vi "Path2PathSup.vi"(8 "Jump Speed":dbl, 9 "Mark Speed":dbl, 10 "Power":dbl, 11 "Combined":T2) -> (3 "PathSupreme":T3)   [LabVIEW 2014]
uses:
  TypeDefs/PathSupreme.ctl
  PBFAM/Controller/MachineController/Converters/ScanSub/VelocityProfile.ctl
  PBFAM/Controller/MachineController/Converters/ScanSub/PathCut.ctl
  PBFAM/Controller/MachineController/Converters/ScanSub/Segment.ctl
  TypeDefs/Point2DwSlope.ctl
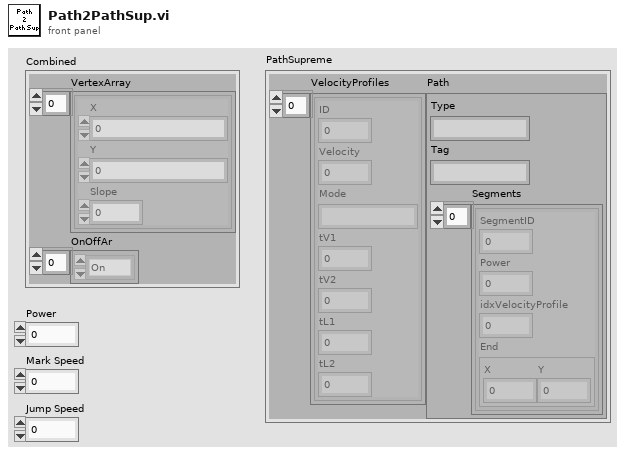
[diagram p1: front panel]
types:
  T1 = typedef "Point2DwSlope.ctl" = cluster{"X":sgl, "Y":sgl, "Slope":dbl}
  T2 = cluster{"VertexArray":T1[], "OnOffAr":enum16{"On", "Off"}[]}
  T3 = typedef "PathSupreme.ctl" = cluster{"VelocityProfiles":T4[], "Path":T5}
  T4 = typedef "VelocityProfile.ctl" = cluster{"ID":u32, "Velocity":dbl, "Mode":string, "tV1":u32, "tV2":u32, "tL1":u32, "tL2":u32}
  T5 = typedef "PathCut.ctl" = cluster{"Type":string, "Tag":string, "Segments":T6[]}
  T6 = typedef "Segment.ctl" = cluster{"SegmentID":u16, "Power":sgl, "idxVelocityProfile":u16, "End":cluster{"X":sgl, "Y":sgl}}
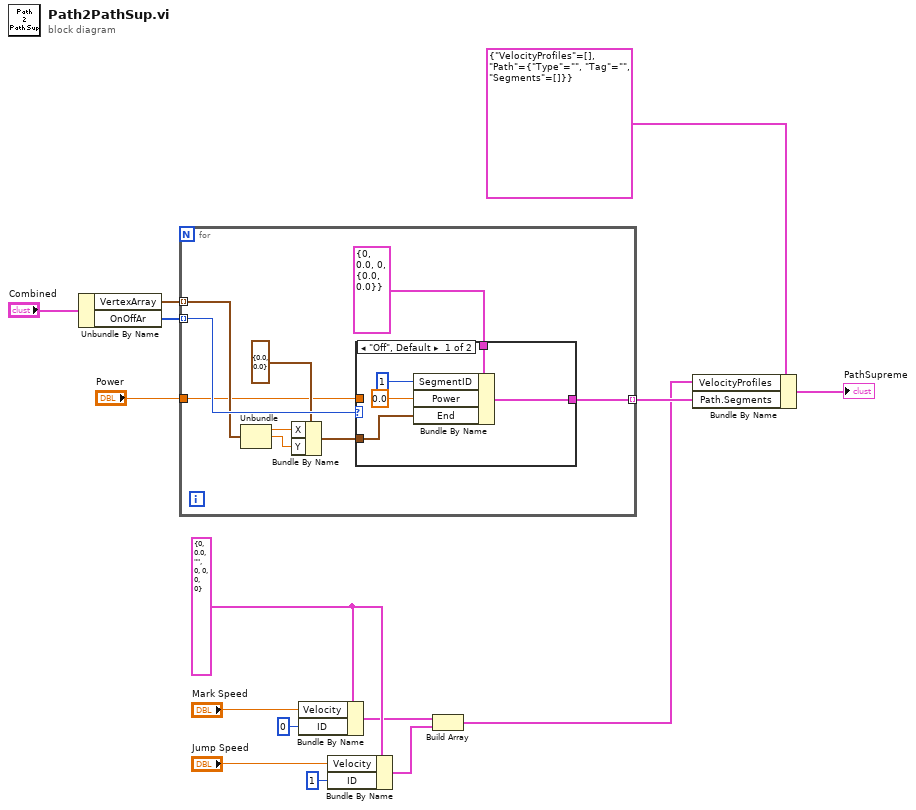
[diagram p0: block diagram]
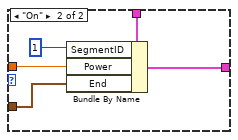
[diagram p2: hidden frame]
diagram:
  w10 = T4 {"ID"=0, "Velocity"=0.0, "Mode"="", "tV1"=0, "tV2"=0, "tL1"=0, "tL2"=0} ("VelocityProfile")
  n1 = Unbundle By Name("Combined") -> ("VertexArray"=w14:T1[], "OnOffAr"=w13:enum16{"On", "Off"}[])
  n2 = for {
    tunnel: w14 -> [w22] mode=indexing
    tunnel: w13 -> [w23] mode=indexing
    tunnel: [w17] -> w3 mode=indexing
    tunnel: "Power" -> [w16]
    n3 = Unbundle(w22) -> ("X"=w20:sgl, "Y"=w19:sgl)  [unwired: 1 out]
    n4 = Bundle By Name(cluster=cluster{"X":sgl, "Y":sgl} {"X"=0.0, "Y"=0.0} ("End"), "X"=w20, "Y"=w19) -> (w18:cluster{"X":sgl, "Y":sgl})
    n5 = case shown="\"Off\", Default" w23 {
      tunnel: T6 {"SegmentID"=0, "Power"=0.0, "idxVelocityProfile"=0, "End"={"X"=0.0, "Y"=0.0}} ("Segment") -> [w29 w34]
      tunnel: w18 -> [w26 w32]
      tunnel: [w25 w31] -> w17
      tunnel: w16 -> [_ w30]
      frame "Off", Default {
        n6 = Bundle By Name(cluster=w29, "SegmentID"=u16 1, "Power"=sgl 0.0, "End"=w26) -> (w25:T6)
      }
      frame "On" {
        n7 = Bundle By Name(cluster=w34, "SegmentID"=u16 1, "Power"=w30, "End"=w32) -> (w31:T6)
      }
    }
  }
  n8 = Bundle By Name(cluster=w10, "Velocity"="Mark Speed", "ID"=u32 0) -> (w7:T4)
  n9 = Bundle By Name(cluster=w10, "Velocity"="Jump Speed", "ID"=u32 1) -> (w6:T4)
  n10 = Build Array(w7, w6) -> (w2:T4[])
  n11 = Bundle By Name(cluster=T3 {"VelocityProfiles"=[], "Path"={"Type"="", "Tag"="", "Segments"=[]}} ("PathSupreme"), "VelocityProfiles"=w2, "Path.Segments"=w3) -> (→"PathSupreme":T3)
